vi "MJG_StageHoming_v2.vi"(8 "error in":errorcluster, 11 "FPGA VI Reference In":refnum<k20>) -> (0 "error out":errorcluster, 2 "XYZ Offsets [enc cnts]":i32[](array[numeric]), 3 "FPGA VI Reference Out":refnum<k20>)   [LabVIEW 2016]
uses:
  <vilib>/rvi/interface/nirviReadWriteControl/nirviReadWriteControl.xnode
  MJG/Subsystems/GLOBALVARS.vi
  IRISS_FPGA_IO.vi
  <vilib>/rvi/errors/niLvFpgaAdjustHostInterfaceError.vi
  FPGA Bitfiles/PhantomControlPI_FPGATarget_QuadCtr2_E2412E44.lvbitx
  <vilib>/rvi/errors/niLvFpgaMergeErrorWithErrorCode.vi
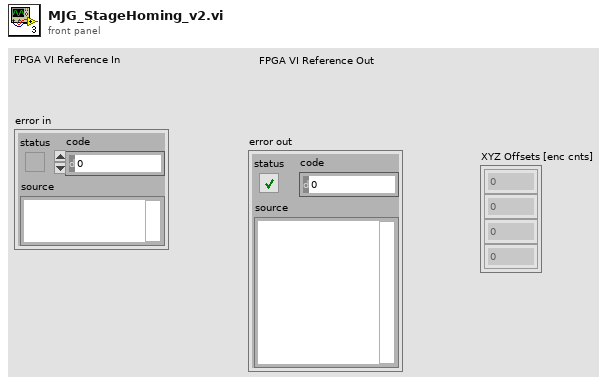
[diagram p1: front panel]
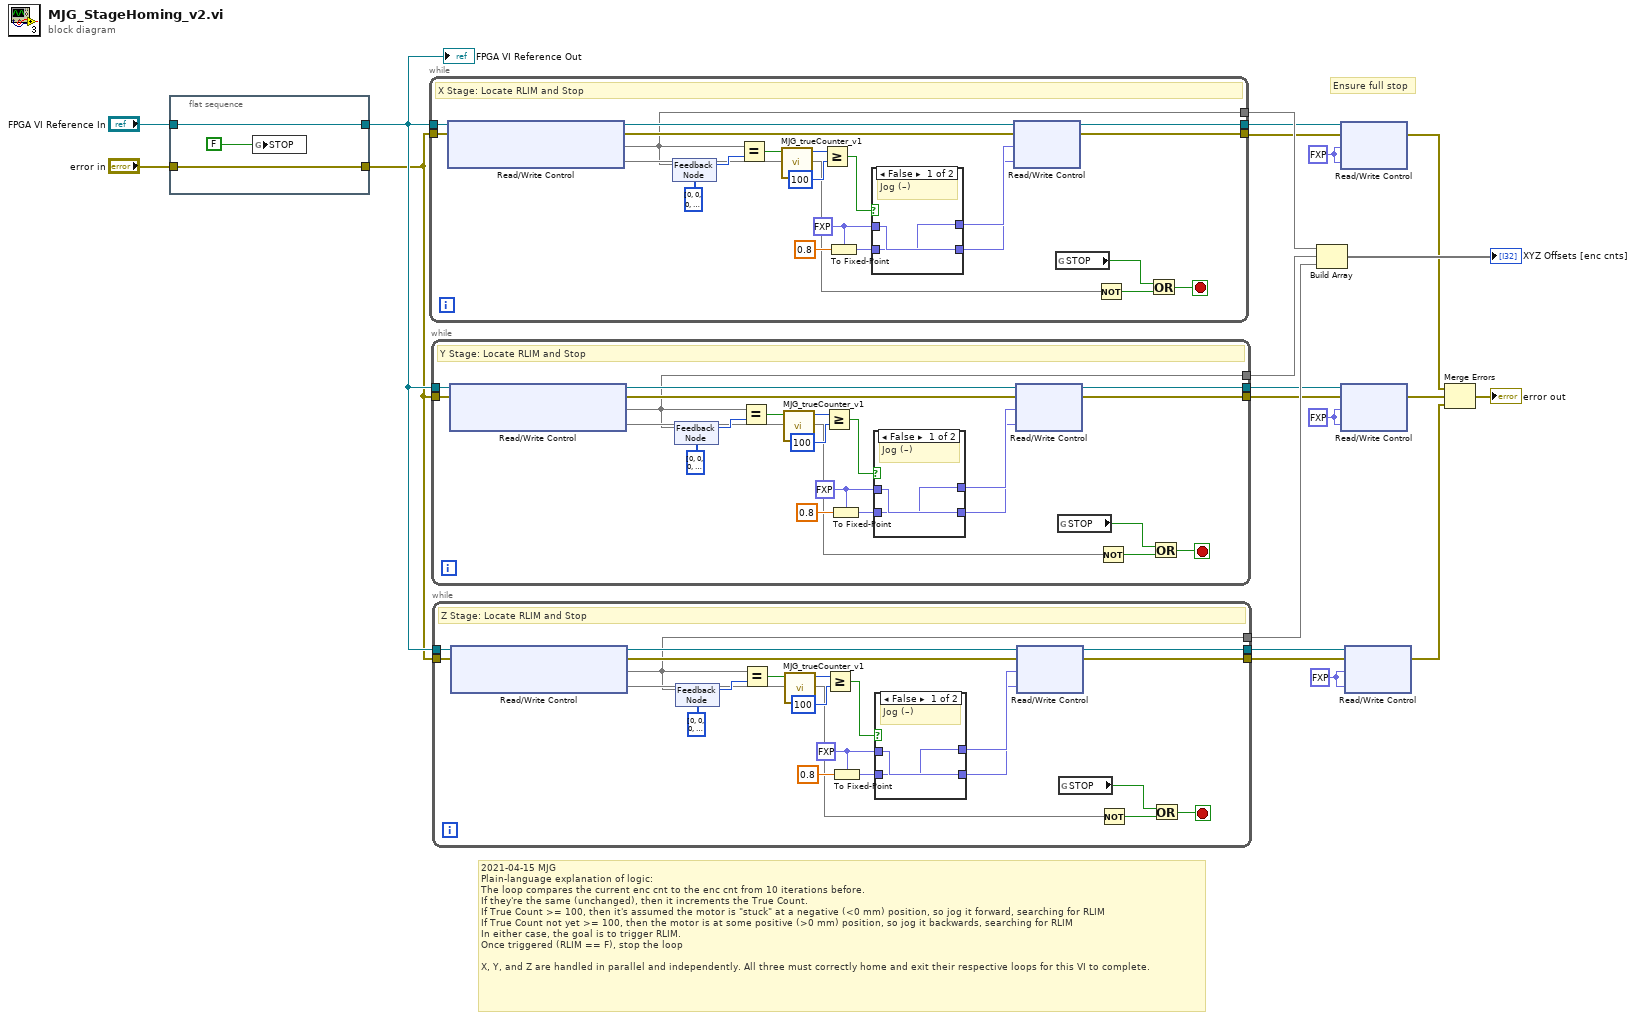
[diagram p0: block diagram]
diagram:
  w14 = fxp<+,32,0> 0.0 ("X PWM 1")
  w13 = fxp<+,32,0> 0.0 ("X PWM 1")
  w17 = fxp<+,32,0> 0.0 ("X PWM 1")
  # "2021-04-15 MJG\nPlain-language explanation of logic:\nThe loop compares the current enc cnt to the enc cnt from 10 iterations before. \nIf they're the same (unchanged), then it increments the True Count.\nIf True Count >= 100, then it's assumed the motor is \"stuck\" at a negative (<0 mm) position, so jog it forward, searching for RLIM\nIf True Count not yet >= 100, then the motor is at some positive (>0 mm) position, so jog it backwards, searching for RLIM\nIn either case, the goal is to trigger RLIM. \nOnce triggered (RLIM == F), stop the loop\n\nX, Y, and Z are handled in parallel and independently. All three must correctly home and exit their respective loops for this VI to complete."
  # "Ensure full stop"
  n1 = flat-sequence {
    tunnel: "FPGA VI Reference In" -> [w23]
    tunnel: "error in" -> [w24]
    tunnel: [w24] -> w1
    tunnel: [w23] -> w2
    frame #0 {
      n2 = global write "GLOBALVARS.vi" "STOP"(FALSE ("program stop")) -> ()
    }
  }
  n3 = while {
    tunnel: w2 -> [w46]
    tunnel: w1 -> [w45]
    tunnel: [w27] -> w20
    tunnel: [w26] -> w15
    tunnel: [w25] -> w16
    stop <- w28 stop-if-true
    w36 = fxp<+,32,0> 0.0 ("X PWM 2")
    # "X Stage: Locate RLIM and Stop"
    n4 = xnode "Read/Write Control"("FPGA VI Reference In"=w46, "error in"=w45) -> ("FPGA VI Reference Out"=w33:refnum<k20>, "error out"=w32:errorcluster, "X Stage Enc Count"=w27, "X Stage RLIM (CONN2/DIO32)"=w31)
    n5 = feedback-in #1(w27) -> ()
    n6 = feedback #1(i32[] [0, 0, 0, 0, 0, 0, 0, 0, 0, 0]) -> (w43:i32)
    n7 = Equal?(x=w27, y=w43) -> (x = y?=w42:bool)
    n8 = call "MJG_trueCounter_v1.vi"("True?"=w42) -> ("True Count"=w41:u32)  [unwired: 10 in]
    n9 = Greater Or Equal?(x=w41, y=u32 100) -> (x >= y?=w38:bool)
    n10 = To Fixed-Point(fixed-point type=w36, number=0.8 ("y")) -> (fixed-point=w37:fxp<+,32,0>)
    n11 = case shown="False" w38 {
      tunnel: w37 -> [w47 w49]
      tunnel: w36 -> [w48 w50]
      tunnel: [w47 w50] -> w35
      tunnel: [w48 w49] -> w34
      frame False {
        # "Jog (–)"
      }
      frame True {
        # "Jog (+)"
      }
    }
    n12 = xnode "Read/Write Control"("FPGA VI Reference In"=w33, "error in"=w32, "X PWM 1"=w35, "X PWM 2"=w34) -> ("FPGA VI Reference Out"=w25:refnum<k20>, "error out"=w26:errorcluster)
    n13 = global read "GLOBALVARS.vi" "STOP"() -> (w30:bool)
    n14 = Not(x=w31) -> (.not. x?=w29:bool)
    n15 = Or(x=w30, y=w29) -> (x .or. y?=w28:bool)
  }
  n16 = while {
    tunnel: w2 -> [w72]
    tunnel: w1 -> [w71]
    tunnel: [w53] -> w19
    tunnel: [w52] -> w11
    tunnel: [w51] -> w12
    stop <- w54 stop-if-true
    w62 = fxp<+,32,0> 0.0 ("X PWM 2")
    # "Y Stage: Locate RLIM and Stop"
    n17 = xnode "Read/Write Control"("FPGA VI Reference In"=w72, "error in"=w71) -> ("FPGA VI Reference Out"=w59:refnum<k20>, "error out"=w58:errorcluster, "Y Stage Enc Count"=w53, "Y Stage RLIM (CONN2/DIO35)"=w57)
    n18 = feedback-in #2(w53) -> ()
    n19 = feedback #2(i32[] [0, 0, 0, 0, 0, 0, 0, 0, 0, 0]) -> (w69:i32)
    n20 = Equal?(x=w53, y=w69) -> (x = y?=w68:bool)
    n21 = call "MJG_trueCounter_v1.vi"("True?"=w68) -> ("True Count"=w67:u32)  [unwired: 10 in]
    n22 = Greater Or Equal?(x=w67, y=u32 100) -> (x >= y?=w64:bool)
    n23 = To Fixed-Point(fixed-point type=w62, number=0.8 ("y")) -> (fixed-point=w63:fxp<+,32,0>)
    n24 = case shown="False" w64 {
      tunnel: w63 -> [w73 w75]
      tunnel: w62 -> [w74 w76]
      tunnel: [w73 w76] -> w61
      tunnel: [w74 w75] -> w60
      frame False {
        # "Jog (–)"
      }
      frame True {
        # "Jog (+)"
      }
    }
    n25 = xnode "Read/Write Control"("FPGA VI Reference In"=w59, "error in"=w58, "Y PWM 1"=w61, "Y PWM 2"=w60) -> ("FPGA VI Reference Out"=w51:refnum<k20>, "error out"=w52:errorcluster)
    n26 = global read "GLOBALVARS.vi" "STOP"() -> (w56:bool)
    n27 = Not(x=w57) -> (.not. x?=w55:bool)
    n28 = Or(x=w56, y=w55) -> (x .or. y?=w54:bool)
  }
  n29 = while {
    tunnel: w2 -> [w98]
    tunnel: w1 -> [w97]
    tunnel: [w79] -> w18
    tunnel: [w78] -> w9
    tunnel: [w77] -> w10
    stop <- w80 stop-if-true
    w88 = fxp<+,32,0> 0.0 ("X PWM 2")
    # "Z Stage: Locate RLIM and Stop"
    n30 = xnode "Read/Write Control"("FPGA VI Reference In"=w98, "error in"=w97) -> ("FPGA VI Reference Out"=w85:refnum<k20>, "error out"=w84:errorcluster, "Z Stage Enc Count"=w79, "Z Stage RLIM (CONN2/DIO38)"=w83)
    n31 = feedback-in #3(w79) -> ()
    n32 = feedback #3(i32[] [0, 0, 0, 0, 0, 0, 0, 0, 0, 0]) -> (w95:i32)
    n33 = Equal?(x=w79, y=w95) -> (x = y?=w94:bool)
    n34 = call "MJG_trueCounter_v1.vi"("True?"=w94) -> ("True Count"=w93:u32)  [unwired: 10 in]
    n35 = Greater Or Equal?(x=w93, y=u32 100) -> (x >= y?=w90:bool)
    n36 = To Fixed-Point(fixed-point type=w88, number=0.8 ("y")) -> (fixed-point=w89:fxp<+,32,0>)
    n37 = case shown="False" w90 {
      tunnel: w89 -> [w99 w101]
      tunnel: w88 -> [w100 w102]
      tunnel: [w99 w102] -> w87
      tunnel: [w100 w101] -> w86
      frame False {
        # "Jog (–)"
      }
      frame True {
        # "Jog (+)"
      }
    }
    n38 = xnode "Read/Write Control"("FPGA VI Reference In"=w85, "error in"=w84, "Z PWM 1"=w87, "Z PWM 2"=w86) -> ("FPGA VI Reference Out"=w77:refnum<k20>, "error out"=w78:errorcluster)
    n39 = global read "GLOBALVARS.vi" "STOP"() -> (w82:bool)
    n40 = Not(x=w83) -> (.not. x?=w81:bool)
    n41 = Or(x=w82, y=w81) -> (x .or. y?=w80:bool)
  }
  n42 = Build Array(w20, w19, w18) -> (→"XYZ Offsets [enc cnts]":void[])
  n43 = xnode "Read/Write Control"("FPGA VI Reference In"=w16, "error in"=w15, "X PWM 1"=w17, "X PWM 2"=w17) -> ("error out"=w8:errorcluster)  [unwired: 1 out]
  n44 = xnode "Read/Write Control"("FPGA VI Reference In"=w12, "error in"=w11, "Y PWM 1"=w13, "Y PWM 2"=w13) -> ("error out"=w7:errorcluster)  [unwired: 1 out]
  n45 = xnode "Read/Write Control"("FPGA VI Reference In"=w10, "error in"=w9, "Z PWM 1"=w14, "Z PWM 2"=w14) -> ("error out"=w6:errorcluster)  [unwired: 1 out]
  n46 = Merge Errors(w8, w7, w6) -> (→"error out":errorcluster)
  "FPGA VI Reference Out" <- w2
